vi "SeCrTS-DD globals.vi"() -> ()   [LabVIEW 2022 SP3]
panel:
  out "Backlog Pump":i32
  out "Backlog Storage":i32
  out "connection ID":refnum<k5>
  out "Storage con?":bool
  in  "writer_Storage":refnum<k21>
  in  "reader_Storage":refnum<k21>
  in  "IP Storage":string="169.254.92.110"
  in  "Log period":dbl
  out "Continuous ?":bool
  in  "IP Pumb":string="169.254.92.110"
  in  "reader_pumb":refnum<k21>
  out "Pumb con?":bool
  in  "writer_Pumb":refnum<k21>
  out "Exit":bool
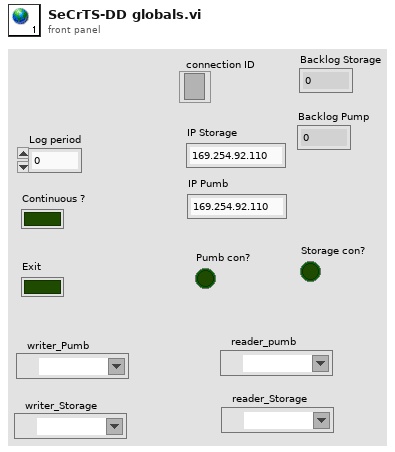
[diagram p1: front panel]
diagram:
